vi "Parameter Cluster To String Cluster.vi"(10 "parameter":T2={"name"="", "direction"=enum."Rx", "default value"=0.0, "unit"="", "Parameter"={"start index"=0, "size"=1, "encoding"=enum."BNR", "signed"=FALSE, "scale multiplier"=1.0, "scale offset"=0.0}}) -> (2 "parameter strings":T1)   [LabVIEW 2020, in "Ballard ARINC 429 System Explorer.lvlib" / "Implementation.lvlib"]
uses:
  Implementation.lvlib
  Shared/VS Channel Definition for Parameter.ctl
  Shared/Direction.ctl
  Shared/Parameter Definition.ctl
  Encoding and Decoding/Encoding.ctl
  Types/Parameter Strings.ctl
  Encoding and Decoding/Encoding and Decoding.lvlib
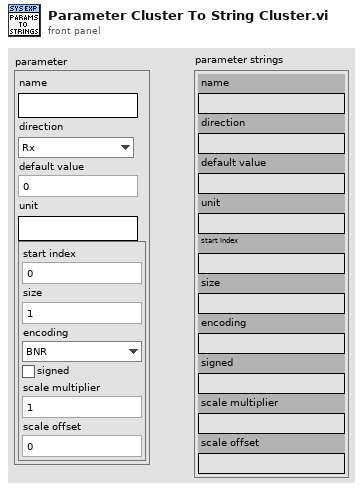
[diagram p1: front panel]
types:
  T1 = typedef "Ballard ARINC 429 System Explorer.lvlib/Implementation.lvlib/Parameter Strings.ctl" = cluster{"name":string, "direction":string, "default value":string, "unit":string, "start index":string, "size":string, "encoding":string, "signed":string, "scale multiplier":string, "scale offset":string}
  T2 = typedef "VS Channel Definition for Parameter.ctl" = cluster{"name":string, "direction":T3, "default value":dbl, "unit":string, "Parameter":T4}
  T3 = typedef "Direction.ctl" = enum16{"Rx", "Tx"}
  T4 = typedef "Parameter Definition.ctl" = cluster{"start index":i32, "size":i32, "encoding":T5, "signed":bool, "scale multiplier":dbl, "scale offset":dbl}
  T5 = typedef "Encoding and Decoding.lvlib/Encoding.ctl" = enum16{"BNR", "BCD", "Discrete"}
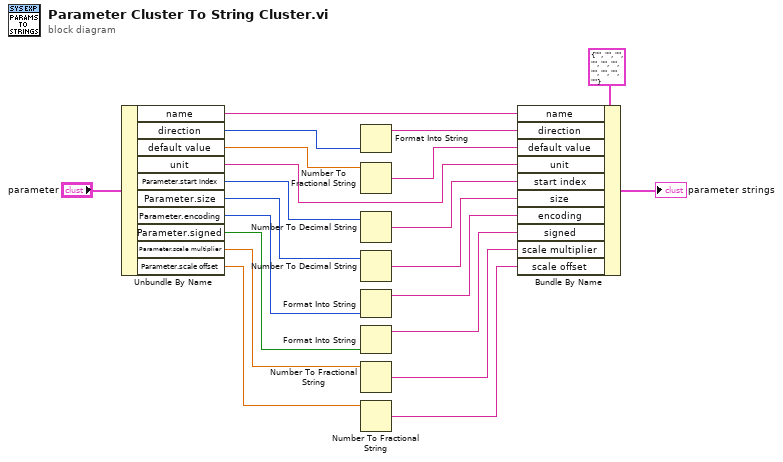
[diagram p0: block diagram]
diagram:
  n1 = Unbundle By Name("parameter") -> ("name"=w18:string, "direction"=w17:T3, "default value"=w15:dbl, "unit"=w13:string, "Parameter.start index"=w12:i32, "Parameter.size"=w11:i32, "Parameter.encoding"=w8:T5, "Parameter.signed"=w1:bool, "Parameter.scale multiplier"=w7:dbl, "Parameter.scale offset"=w6:dbl)
  n2 = Format Into String(w17) -> (resulting string=w16:string)  [unwired: 3 in, 1 out]
  n3 = Number To Fractional String(number=w15) -> (F-format string=w14:string)  [unwired: 3 in]
  n4 = Number To Decimal String(number=w12) -> (decimal integer string=w10:string)  [unwired: 1 in]
  n5 = Number To Decimal String(number=w11) -> (decimal integer string=w9:string)  [unwired: 1 in]
  n6 = Format Into String(w8) -> (resulting string=w3:string)  [unwired: 3 in, 1 out]
  n7 = Format Into String(w1) -> (resulting string=w2:string)  [unwired: 3 in, 1 out]
  n8 = Number To Fractional String(number=w7) -> (F-format string=w5:string)  [unwired: 3 in]
  n9 = Number To Fractional String(number=w6) -> (F-format string=w4:string)  [unwired: 3 in]
  n10 = Bundle By Name(cluster=T1 {"name"="", "direction"="", "default value"="", "unit"="", "start index"="", "size"="", "encoding"="", "signed"="", "scale multiplier"="", "scale offset"=""} ("parameter strings"), "name"=w18, "direction"=w16, "default value"=w14, "unit"=w13, "start index"=w10, "size"=w9, "encoding"=w3, "signed"=w2, "scale multiplier"=w5, "scale offset"=w4) -> (→"parameter strings":T1)
